vi "CFTS-Check State.vi"(8 "error in (no error)":errorcluster, 11 "Expt State":T1) -> (0 "error out":errorcluster)   [LabVIEW 2020]
uses:
  CFTS-Experiment State.ctl
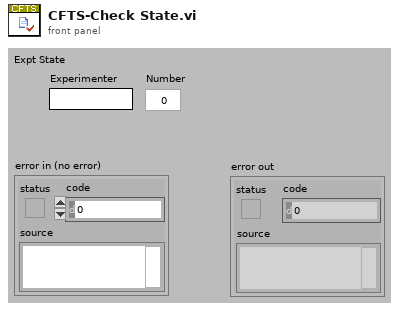
[diagram p1: front panel]
types:
  T1 = typedef "CFTS-Experiment State.ctl" = cluster{"Experimenter":string, "Number":u32, "Right":string, "Left":string, "Data Folder":path, "State File":path, "Version Info":string, "End Exposure Time":dbl, "Exposure Duration":string, "Run #":cluster{"CAP":i16, "ABR":i16, "DP":i16, "VsEP":i16, "MeasSeq":i16, "SubSeq":i16, "SFOAE":i16}}
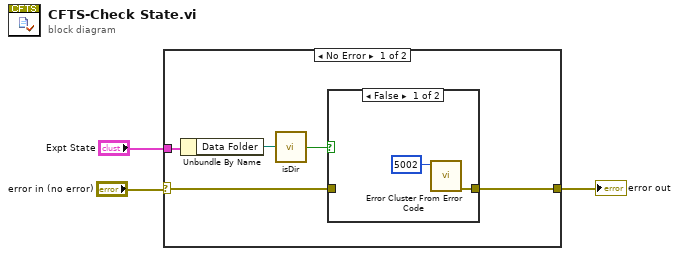
[diagram p0: block diagram]
diagram:
  n1 = case shown="No Error" "error in (no error)" {
    selector: "error in (no error)" -> [w5 w12]
    tunnel: [w4 w12] -> w2
    tunnel: "Expt State" -> [w8 _]
    frame No Error {
      n2 = Unbundle By Name(w8) -> ("Data Folder"=w7:path)
      n3 = call "isDir.vi"("path"=w7) -> ("is Dir?"=w6:bool)
      n4 = case shown="False" w6 {
        tunnel: w5 -> [_ w11]
        tunnel: [w10 w11] -> w4
        frame False {
          n5 = call <vilib>:"Error Cluster From Error Code.vi"("error code (0)"=5002) -> ("error out"=w10:errorcluster)  [unwired: 8 in]
        }
        frame True {
        }
      }
    }
    frame Error {
    }
  }
  "error out" <- w2
